vi "Analysis Configuration Dialog.vi"(11 "Data In":T1={"UI References"={"Exit Ref"=refnum, "Save Ref"=refnum, "Open Ref"=refnum, "Export Ref"=refnum, "Acquire Ref"=refnum, "Configure Ref"=refnum, "Graph Ref"=refnum, "Clear Ref"=refnum, "Analyze Ref"=refnum, "Status Ref"=refnum, "Snapshot Ref"=refnum, "Network Ref"=refnum, "Timeslice Ref"=refnum, "DAQSetting Ref"=refnum, "SystemSet"=refnum, "Path ref"=refnum, "Data OK Ref"=refnum}, "Graph Data"={"Data"=[], "Annotation List"=[], "Cursor List"=[], "Analysis Data"=[]}, "User Specified"={"Hardware Configuration"={"HW Refnum <Replace Me>"="", "Signal Type <Replace Me>"=enum."Sine Wave"}, "Analysis Configuration"={"Statistics"=TRUE}, "New Data Behavior"=enum."Replace", "Aspic Seeting"={"Gain"=0, "RC"=0, "aspic1Data"=[], "aspic2Data"=[], "AF1"=FALSE, "Mode"=enum."TM"}, "Network"={"invert_send"=TRUE, "Number of datagrams to read"=5000, "max bytes/read"=2500, "Timeout"=4000, "host"="192.168.1.18", "Port Receive"=5678}, "timeslice"={"Time slice"=[], "Durations"=[], "names of control"=[]}, "Acquisition Settings"={"pixel number"=0, "repetition"=0, "Trigger"=enum."Ethernet via Labview"}, "CommSelect"=enum."resetFifo18ASPIC", "Path"={"TS file"=path "C:/Users/lpnhe/Desktop/Labview/damic/DAMIC-LTC/DamicLTC-seul-Essai.txt", "Log file"=path "C:/DAMIC/DAMIC-LTC/Data/log.txt", "Log Directory"=path "C:/DAMIC/DAMIC-LTC/Data", "Output aspic file folder"=path "C:/Users/lpnhe/Desktop/Labview/damic/DAMIC-LTC/Data", "TSfile folder"=path "C:/Users/lpnhe/Desktop/Labview/damic/DAMIC_TIMESLICE"}}, "System Set"=FALSE, "Results"={"Max"=[], "Min"=[], "Average"=[], "S.D"=[], "Variance"=[]}, "Data OK"=FALSE} {"User Specified"."Network"."Number of datagrams to read" format="%0d"}) -> (3 "Data out":T1={"UI References"={"Exit Ref"=refnum, "Save Ref"=refnum, "Open Ref"=refnum, "Export Ref"=refnum, "Acquire Ref"=refnum, "Configure Ref"=refnum, "Graph Ref"=refnum, "Clear Ref"=refnum, "Analyze Ref"=refnum, "Status Ref"=refnum, "Snapshot Ref"=refnum, "Network Ref"=refnum, "Timeslice Ref"=refnum, "DAQSetting Ref"=refnum, "SystemSet"=refnum, "Path ref"=refnum, "Data OK Ref"=refnum}, "Graph Data"={"Data"=[], "Annotation List"=[], "Cursor List"=[], "Analysis Data"=[]}, "User Specified"={"Hardware Configuration"={"HW Refnum <Replace Me>"="", "Signal Type <Replace Me>"=enum."Sine Wave"}, "Analysis Configuration"={"Statistics"=TRUE}, "New Data Behavior"=enum."Replace", "Aspic Seeting"={"Gain"=0, "RC"=0, "aspic1Data"=[], "aspic2Data"=[], "AF1"=FALSE, "Mode"=enum."TM"}, "Network"={"invert_send"=TRUE, "Number of datagrams to read"=5000, "max bytes/read"=2500, "Timeout"=4000, "host"="192.168.1.18", "Port Receive"=5678}, "timeslice"={"Time slice"=[], "Durations"=[], "names of control"=[]}, "Acquisition Settings"={"pixel number"=0, "repetition"=0, "Trigger"=enum."Ethernet via Labview"}, "CommSelect"=enum."resetFifo18ASPIC", "Path"={"TS file"=path "C:/Users/lpnhe/Desktop/Labview/damic/DAMIC-LTC/DamicLTC-seul-Essai.txt", "Log file"=path "C:/DAMIC/DAMIC-LTC/Data/log.txt", "Log Directory"=path "C:/DAMIC/DAMIC-LTC/Data", "Output aspic file folder"=path "C:/Users/lpnhe/Desktop/Labview/damic/DAMIC-LTC/Data", "TSfile folder"=path "C:/Users/lpnhe/Desktop/Labview/damic/DAMIC_TIMESLICE"}}, "System Set"=FALSE, "Results"={"Max"=[], "Min"=[], "Average"=[], "S.D"=[], "Variance"=[]}, "Data OK"=FALSE} {"User Specified"."Network"."Number of datagrams to read" format="%0d"})   [LabVIEW 2014]
doc: "Displays the analysis configuration dialog if the user has the \"Prompt?\" preference set."
uses:
  controls/Data.ctl
  controls/UI References.ctl
  controls/Data OK.ctl
  controls/Graph Data.ctl
  <vilib>/Utility/miscctls.llb/LVAnnotationListTypeDef.ctl
  <vilib>/Utility/miscctls.llb/LVCursorListTypeDef.ctl
  controls/User Specified Data.ctl
  controls/HW Configuration.ctl
  controls/Simulated Signal Type.ctl
  controls/Analysis Configuration.ctl
  controls/New Data Behavior.ctl
  controls/AspicSettings.ctl
  controls/AspicMode.ctl
  controls/Network.ctl
  controls/Timeslice.ctl
  controls/DAQSettings.ctl
  controls/TriggerMode.ctl
  controls/CommSelect.ctl
  common/Comm/path.ctl
  controls/SystemSet.ctl
  common/Comm/analysis.ctl
panel:
  # "(Scroll up to see large state data in/out clusters)"
  # "CH0"
  # "CH1"
  # "CH2"
  # "CH3"
  # "CH4"
  # "CH5"
  # "CH6"
  # "CH7"
  # "CH0"
  # "CH1"
  # "CH2"
  # "CH3"
  # "CH4"
  # "CH5"
  # "CH6"
  # "CH7"
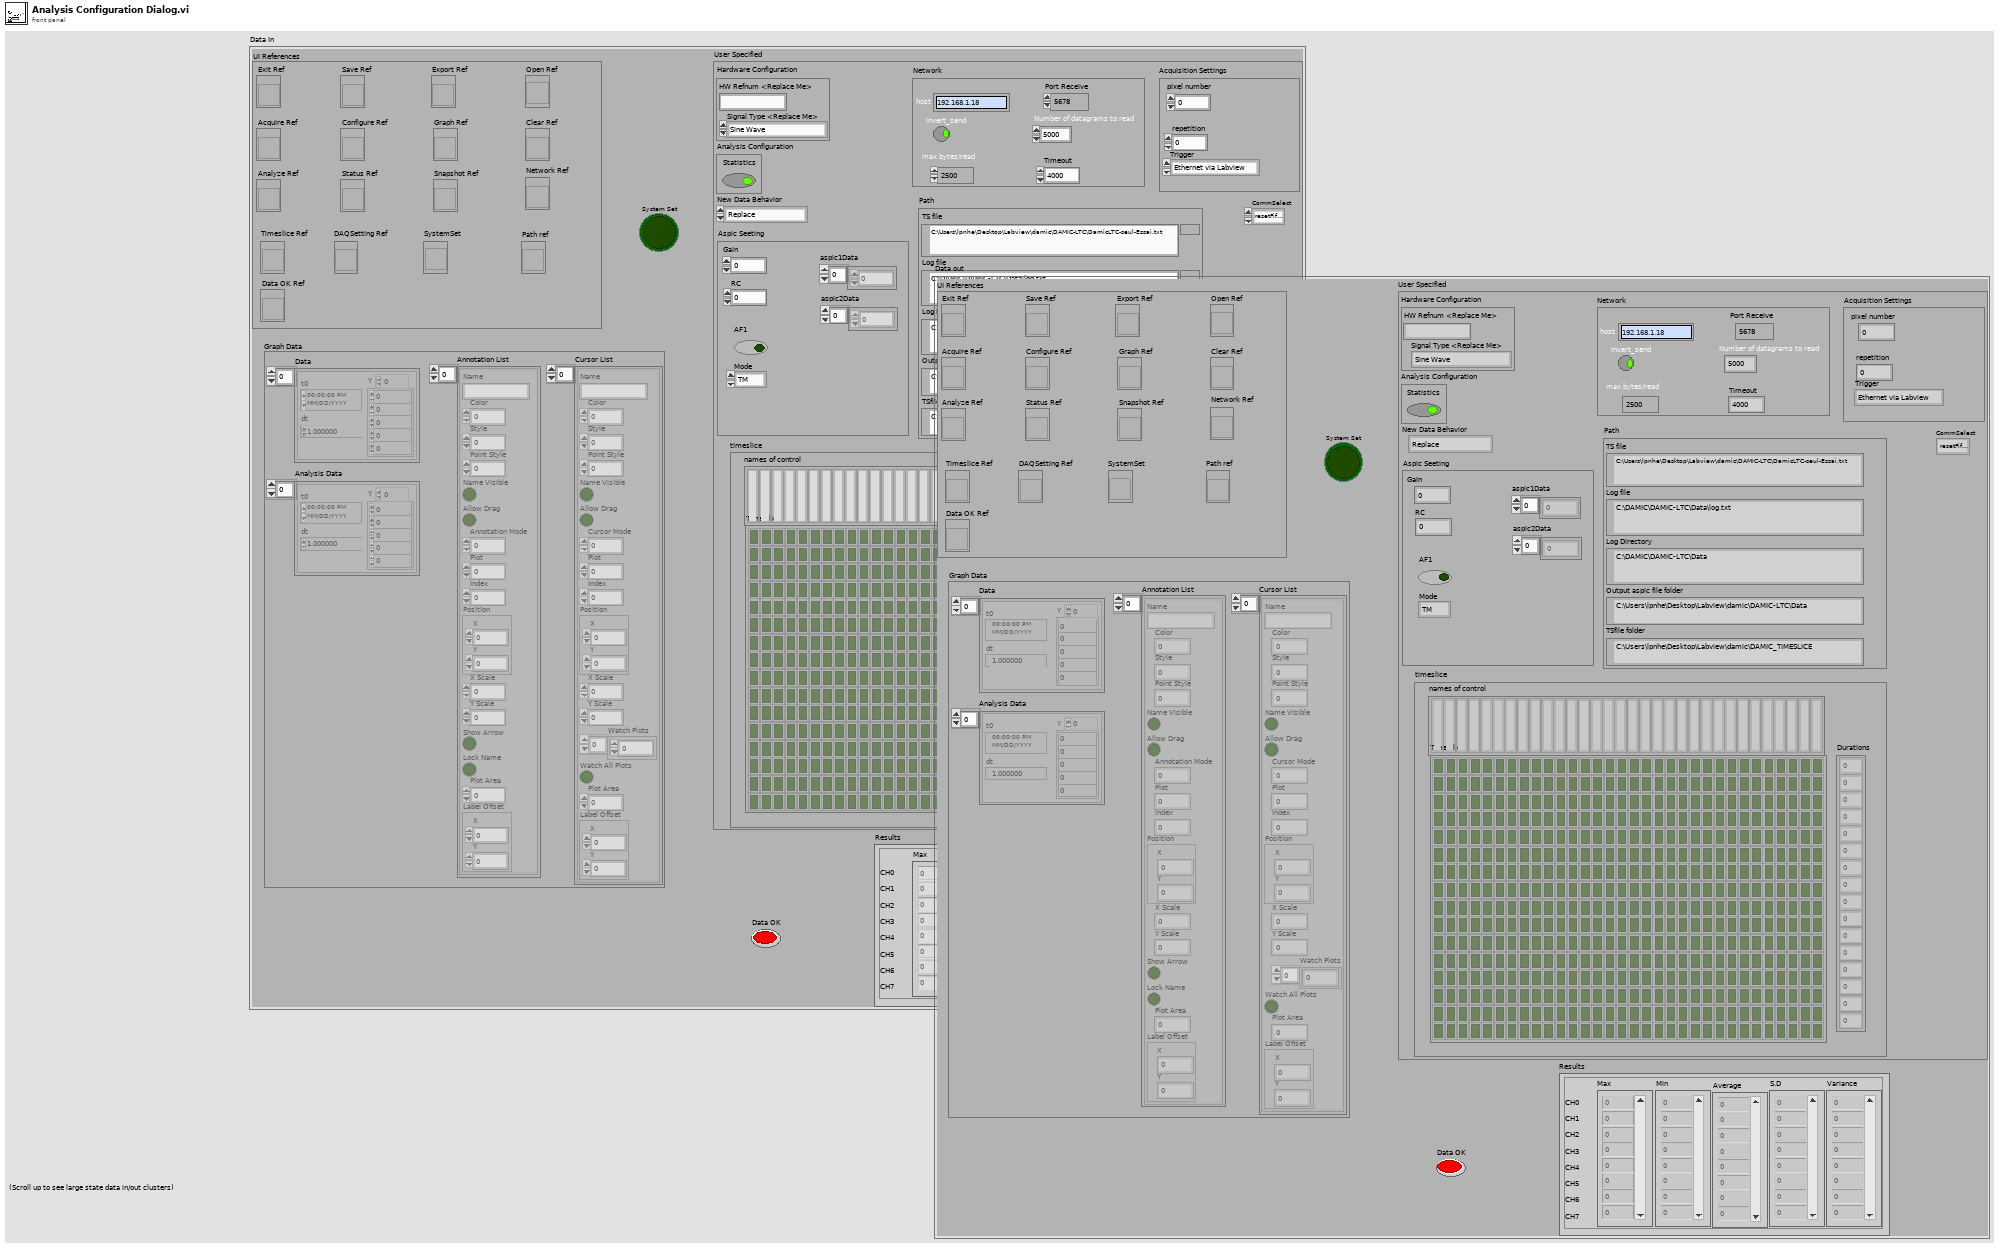
[diagram p1: front panel]
types:
  T1 = typedef "Data.ctl" = cluster{"UI References":T2, "Graph Data":T3, "User Specified":T6, "System Set":T19, "Results":T20, "Data OK":T21}
  T2 = typedef "UI References.ctl" = cluster{"Exit Ref":refnum<vi>, "Save Ref":refnum<vi>, "Open Ref":refnum<vi>, "Export Ref":refnum<vi>, "Acquire Ref":refnum<vi>, "Configure Ref":refnum<vi>, "Graph Ref":refnum<vi>, "Clear Ref":refnum<vi>, "Analyze Ref":refnum<vi>, "Status Ref":refnum<vi>, "Snapshot Ref":refnum<vi>, "Network Ref":refnum<vi>, "Timeslice Ref":refnum<vi>, "DAQSetting Ref":refnum<vi>, "SystemSet":refnum<vi>, "Path ref":refnum<vi>, "Data OK Ref":refnum<vi>}
  T3 = typedef "Graph Data.ctl" = cluster{"Data":waveform(dbl)[], "Annotation List":T4, "Cursor List":T5, "Analysis Data":waveform(dbl)[]}
  T4 = typedef "LVAnnotationListTypeDef.ctl" = cluster{"Name":string, "Color":u32, "Style":u8, "Point Style":u8, "Name Visible":bool, "Allow Drag":bool, "Annotation Mode":u32, "Plot":i32, "Index":i32, "Position":cluster{"X":dbl, "Y":dbl}, "X Scale":u32, "Y Scale":u32, "Show Arrow":bool, "Lock Name":bool, "Plot Area":i32, "Label Offset":cluster{"X":dbl, "Y":dbl}}[]
  T5 = typedef "LVCursorListTypeDef.ctl" = cluster{"Name":string, "Color":u32, "Style":u8, "Point Style":u8, "Name Visible":bool, "Allow Drag":bool, "Cursor Mode":u32, "Plot":i32, "Index":i32, "Position":cluster{"X":dbl, "Y":dbl}, "X Scale":u32, "Y Scale":u32, "Watch Plots":i32[], "Watch All Plots":bool, "Plot Area":i32, "Label Offset":cluster{"X":dbl, "Y":dbl}}[]
  T6 = typedef "User Specified Data.ctl" = cluster{"Hardware Configuration":T7, "Analysis Configuration":T9, "New Data Behavior":T10, "Aspic Seeting":T11, "Network":T13, "timeslice":T14, "Acquisition Settings":T15, "CommSelect":T17, "Path":T18}
  T7 = typedef "HW Configuration.ctl" = cluster{"HW Refnum <Replace Me>":string, "Signal Type <Replace Me>":T8}
  T8 = typedef "Simulated Signal Type.ctl" = enum16{"Sine Wave", "Square Wave"}
  T9 = typedef "Analysis Configuration.ctl" = cluster{"Statistics":bool}
  T10 = typedef "New Data Behavior.ctl" = enum16{"Replace", "Overlay", "Append"}
  T11 = typedef "AspicSettings.ctl" = cluster{"Gain":u8, "RC":u8, "aspic1Data":u32[], "aspic2Data":u32[], "AF1":bool, "Mode":T12}
  T12 = typedef "AspicMode.ctl" = enum16{"DSI", "TM"}
  T13 = typedef "Network.ctl" = cluster{"invert_send":bool, "Number of datagrams to read":u32, "max bytes/read":i32, "Timeout":i32, "host":string, "Port Receive":u16}
  T14 = typedef "Timeslice.ctl" = cluster{"Time slice":bool[][], "Durations":dbl[], "names of control":string[]}
  T15 = typedef "DAQSettings.ctl" = cluster{"pixel number":u32, "repetition":u32, "Trigger":T16}
  T16 = typedef "TriggerMode.ctl" = enum16{"Ethernet via Labview", "SMA (1.8V)"}
  T17 = typedef "CommSelect.ctl" = enum16{"startTSL", "writeCABAC", "readCABAC", "resetCABAC", "emissionTest", "regRead", "executeASPIC", "resetASPIC", "resetFifo18ASPIC", "resetFifo16ASPIC", "LabviewDamicStart"}
  T18 = typedef "path.ctl" = cluster{"TS file":path, "Log file":path, "Log Directory":path, "Output aspic file folder":path, "TSfile folder":path}
  T19 = typedef "SystemSet.ctl" = bool
  T20 = typedef "analysis.ctl" = cluster{"Max":i32[], "Min":i32[], "Average":dbl[], "S.D":dbl[], "Variance":dbl[]}
  T21 = typedef "Data OK.ctl" = bool
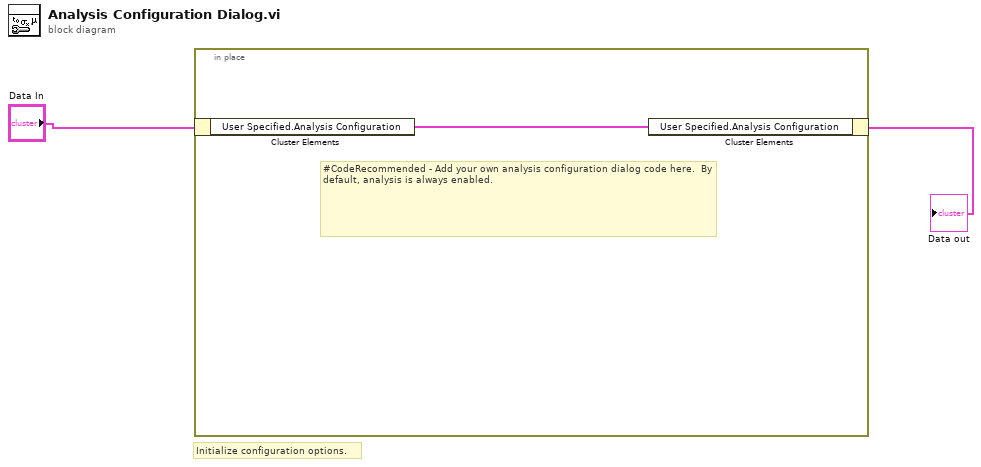
[diagram p0: block diagram]
diagram:
  # "Initialize configuration options."
  n1 = in-place {
    # "#CodeRecommended - Add your own analysis configuration dialog code here.  By default, analysis is always enabled."
    n2 = in-place-cluster #1("Data In") -> ("User Specified.Analysis Configuration"=w3:T9)
    n3 = in-place-cluster #1("User Specified.Analysis Configuration"=w3) -> (→"Data out":T1)
  }
